vi "Load Qualified Path Groups.vi"(0 "Class Files":path[](array[path]), 11 "error in":errorcluster) -> (4 "Path Groups out":refnum<class "Path Group.lvclass">[](array[class]), 15 "error out":errorcluster)   [LabVIEW 2023, in "RFCalAndFixtureCharact.Common.lvlib"]
uses:
  RFCalAndFixtureCharact.Common.lvlib
  Base Classes/Path Group/Path Group.lvclass
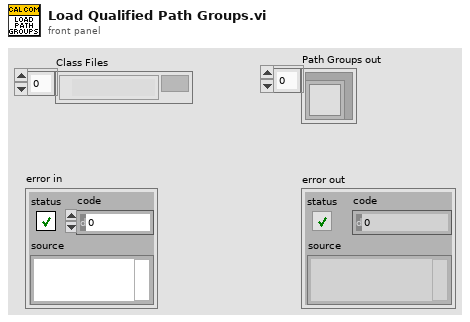
[diagram p1: front panel]
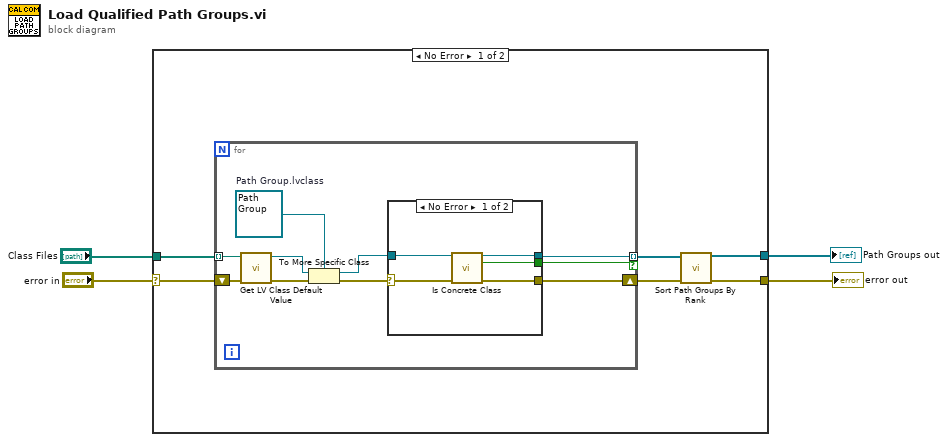
[diagram p0: block diagram]
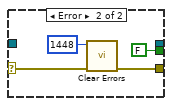
[diagram p2: hidden frame]
diagram:
  n1 = case shown="No Error" "error in" {
    selector: "error in" -> [w6 w30]
    tunnel: "Class Files" -> [w5 _]
    tunnel: [w9 w30] -> w3
    tunnel: [w7 _] -> w2
    frame No Error {
      n2 = for {
        shift-right: [w14] -> w10
        shift-left: w6 -> [w20]
        tunnel: [w13] -> w8 mode=indexing if=w11
        tunnel: w5 -> [w12] mode=indexing
        w17 = refnum<class "Path Group.lvclass"> refnum  # Path Group.lvclass
        n3 = call <vilib>:"Get LV Class Default Value.vi"("error in (no error)"=w20, "class path"=w12) -> ("error out"=w18:errorcluster, "object"=w19:refnum<class>)  [unwired: 8 in]
        n4 = To More Specific Class(target class=w17, reference=w19, error in=w18) -> (specific class reference=w15:refnum<class "Path Group.lvclass">, error out=w16:errorcluster)
        n5 = case shown="No Error" w16 {
          selector: w16 -> [w23 w29]
          tunnel: w15 -> [w25 _]
          tunnel: [w22 w28] -> w14
          tunnel: [w24 _] -> w13
          tunnel: [w21 FALSE ("Is Concrete Class?")] -> w11
          frame No Error {
            n6 = call-dynamic "Is Concrete Class.vi"("Path Group in"=w25, "error in (no error)"=w23) -> ("Path Group out"=w24:refnum<class "Path Group.lvclass">, "Is Concrete Class?"=w21:bool, "error out"=w22:errorcluster)  [unwired: 11 in]
          }
          frame Error {
            n7 = call <vilib>:"Clear Errors.vi"("error in (no error)"=w29, "specific error code to clear (0: all)"=1448) -> ("error out"=w28:errorcluster)  [unwired: 4 in, 1 out]
          }
        }
      }
      n8 = call "Sort Path Groups By Rank.vi"("Path Groups in"=w8, "error in (no error)"=w10) -> ("Path Groups out"=w7:refnum<class "Path Group.lvclass">[], "error out"=w9:errorcluster)  [unwired: 12 in]
    }
    frame Error {
    }
  }
  "error out" <- w3
  "Path Groups out" <- w2
